vi "Parse Property Type.vi"(8 "error in":errorcluster, 11 "Node in":refnum<k20>) -> (0 "error out":errorcluster, 2 "Property Type":T1, 3 "Child Node out":refnum<k20>)   [LabVIEW 2024, in "Parser.lvlib" / "Property.lvclass"]
uses:
  Property.lvclass
  Controls/Property Type.ctl
  <vilib>/xml/Close Reference(Node).vi
  <vilib>/xml/NI_XML.lvlib
  <resource>/objmgr/DOMUserDefRef.rc
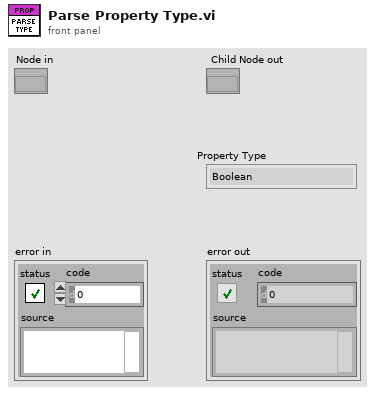
[diagram p1: front panel]
types:
  T1 = typedef "Parser.lvlib/Property.lvclass/Property Type.ctl" = enum16{"Boolean", "Double", "String", "Path", "Dictionary", "DependentFile", "I16", "I32", "I64", "U16", "U32", "U64", "BooleanArray", "DoubleArray", "StringArray", "I16Array", "I32Array", "I64Array", "U16Array", "U32Array", "U64Array", "Variant"}
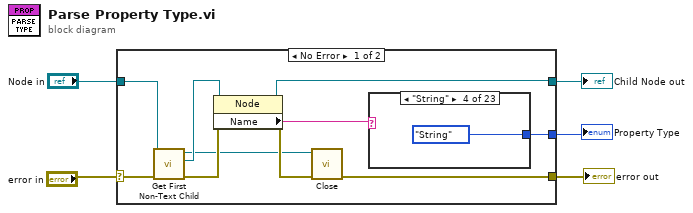
[diagram p0: block diagram]
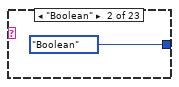
[diagram p3: hidden frame]
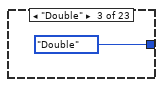
[diagram p4: hidden frame]
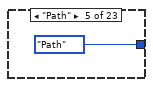
[diagram p5: hidden frame]
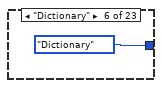
[diagram p6: hidden frame]
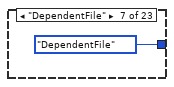
[diagram p7: hidden frame]
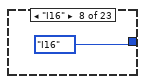
[diagram p8: hidden frame]
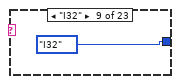
[diagram p9: hidden frame]
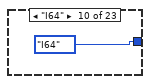
[diagram p10: hidden frame]
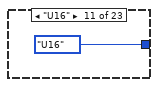
[diagram p11: hidden frame]
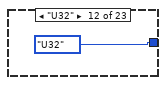
[diagram p12: hidden frame]
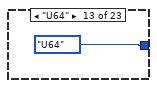
[diagram p13: hidden frame]
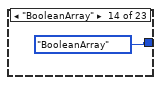
[diagram p14: hidden frame]
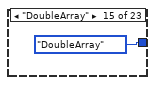
[diagram p15: hidden frame]
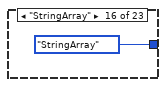
[diagram p16: hidden frame]
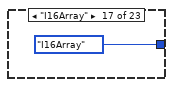
[diagram p17: hidden frame]
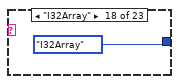
[diagram p18: hidden frame]
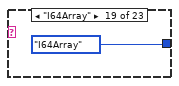
[diagram p19: hidden frame]
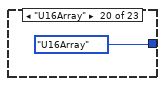
[diagram p20: hidden frame]
diagram:
  n1 = case shown="No Error" "error in" {
    selector: "error in" -> [w12 w39]
    tunnel: [w14 w39] -> w5
    tunnel: [w10 w38] -> w3
    tunnel: "Node in" -> [w9 w38]
    tunnel: [w7 _] -> w1
    frame No Error {
      n2 = call <vilib>:"Get First Non-Text Child.vi"("error in (no error)"=w12, "node in"=w9) -> ("error out"=w15:errorcluster, "child node"=w11:refnum<k20>, "node out"=w8:refnum<k20>)  [unwired: 6 in, 1 out]
      n3 = property on="Property Node" class="Node"(reference=w11, error in=w15) -> (reference out=w10:refnum<k20>, error out=w13:errorcluster, "Name"=w6:string)
      n4 = call-poly <vilib>:"Close.vi"("error in (no error)"=w13, "node"=w8) -> ("error out"=w14:errorcluster)  [unwired: 7 in]
      n5 = case shown="\"String\"" w6 {
        tunnel: [_ Property_Type."Boolean" ("Property Type") Property_Type."Double" ("Property Type") Property_Type."String" ("Property Type") Property_Type."Path" ("Property Type") Property_Type."Dictionary" ("Property Type") Property_Type."DependentFile" ("Property Type") Property_Type."I16" ("Property Type") Property_Type."I32" ("Property Type") Property_Type."I64" ("Property Type") Property_Type."U16" ("Property Type") Property_Type."U32" ("Property Type") Property_Type."U64" ("Property Type") Property_Type."BooleanArray" ("Property Type") Property_Type."DoubleArray" ("Property Type") Property_Type."StringArray" ("Property Type") Property_Type."I16Array" ("Property Type") Property_Type."I32Array" ("Property Type") Property_Type."I64Array" ("Property Type") Property_Type."U16Array" ("Property Type") Property_Type."U32Array" ("Property Type") Property_Type."U64Array" ("Property Type") Property_Type."Variant" ("Property Type")] -> w7
        frame "False" {
        }
        frame "Boolean" {
        }
        frame "Double" {
        }
        frame "String" {
        }
        frame "Path" {
        }
        frame "Dictionary" {
        }
        frame "DependentFile" {
        }
        frame "I16" {
        }
        frame "I32" {
        }
        frame "I64" {
        }
        frame "U16" {
        }
        frame "U32" {
        }
        frame "U64" {
        }
        frame "BooleanArray" {
        }
        frame "DoubleArray" {
        }
        frame "StringArray" {
        }
        frame "I16Array" {
        }
        frame "I32Array" {
        }
        frame "I64Array" {
        }
        frame "U16Array" {
        }
        frame "U32Array" {
        }
        frame "U64Array" {
        }
        frame "Variant", Default {
        }
      }
    }
    frame Error {
    }
  }
  "Child Node out" <- w3
  "error out" <- w5
  "Property Type" <- w1
